vi "Test Roundtrip Serialize Waveforms.vi"(8 "error in (no error)":errorcluster) -> (0 "error out":errorcluster)   [LabVIEW 2013]
uses:
  src/Serializer/JSON Serializer/JSON Serializer.lvclass
  src/Deserializer/JSON Deserializer/JSON Deserializer.lvclass
  <vilib>/addons/_JKI Toolkits/Caraya/classes/Test/Test.lvclass
  <vilib>/addons/_JKI Toolkits/Caraya/classes/Assert/Assert.lvclass
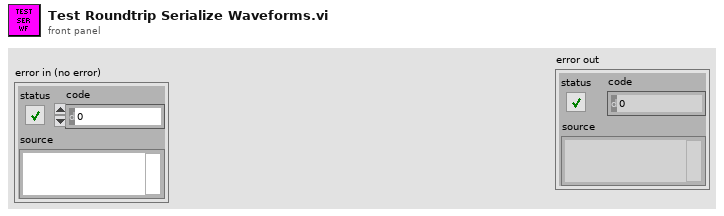
[diagram p1: front panel]
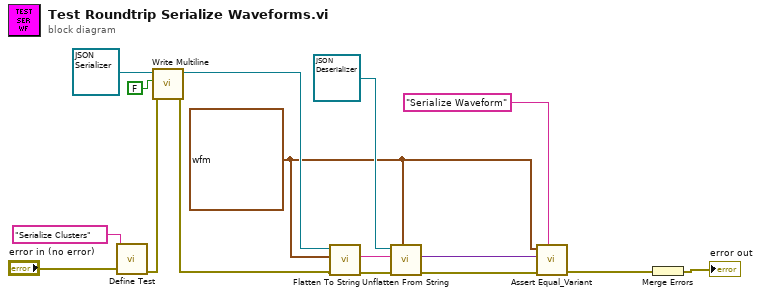
[diagram p0: block diagram]
diagram:
  w2 = waveform(dbl) {"t0"=timestamp(3550405937.679 s since 1904-01-01), "dt"=0.1, "Y"=[1.0, 2.0, 3.0]} ("Waveform")
  n1 = call <vilib>:"Define Test.vi"("error in (no error)"="error in (no error)", "Label (VI Title)"="Serialize Clusters") -> ("error out"=w12:errorcluster)  [unwired: 9 in]
  n2 = call-dynamic "Write Multiline.vi"("error in (no error)"=w12, "Multiline"=FALSE, "JSON Serializer in"=refnum<class "JSON Serializer.lvclass"> refnum ("JKI JSON Serialization.lvlib:JSON Serializer.lvclass")) -> ("error out"=w8:errorcluster, "JSON Serializer out"=w7:refnum<class "JSON Serializer.lvclass">)  [unwired: 7 in]
  n3 = call-dynamic "Flatten To String.vi"("error in (no error)"=w8, "Variant"=w2, "JSON Serializer in"=w7) -> ("error out"=w4:errorcluster, "String"=w5:string)  [unwired: 6 in, 1 out]
  n4 = call-dynamic "Unflatten From String.vi"("Type and Defaults"=w2, "error in (no error)"=w4, "String"=w5, "Deserializer in"=refnum<class "JSON Deserializer.lvclass"> refnum) -> ("error out"=w1:errorcluster, "Variant"=w3:variant)  [unwired: 5 in, 1 out]
  n5 = call <vilib>:"Assert Equal_Variant.vi"("Label"="Serialize Waveform", "error in (no error)"=w1, "Y"=w3, "X"=w2) -> ("error out"=w9:errorcluster)  [unwired: 7 in]
  n6 = Merge Errors(w9) -> (→"error out":errorcluster)
